vi "Disconnect.vi"(7 "error in (no error)":errorcluster, 10 "I-O in":refnum<class "I-O.lvclass">) -> (0 "error out":errorcluster)   [LabVIEW 2019, in "I-O.lvclass"]
uses:
  I-O.lvclass
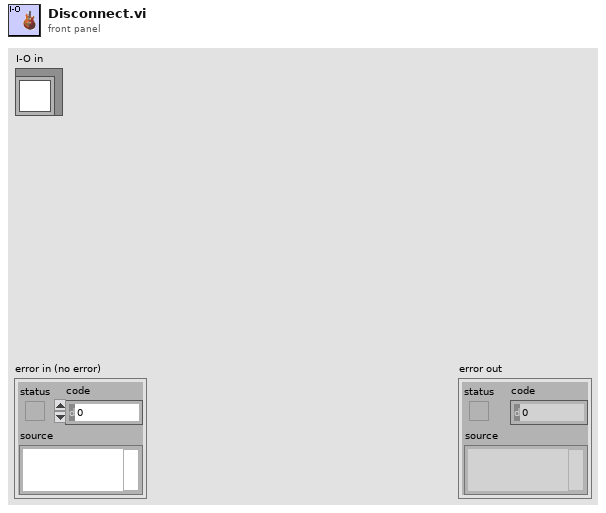
[diagram p1: front panel]
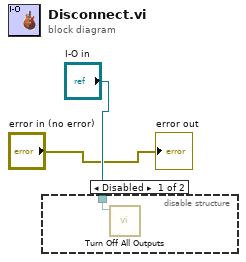
[diagram p0: block diagram]
diagram:
  n1 = disable-structure shown="Disabled" {
    disable-tunnel: "I-O in" -> [w3 _]
    frame Disabled {
      n2 = call-dynamic "Turn Off All Outputs.vi"("I-O in"=w3) -> ()  [unwired: 9 in, 2 out]
    }
    frame Enabled {
    }
  }
  "error out" <- "error in (no error)"
